vi "ReadFile.vi"(1 "Name":string="C:\\Users\\Abhi\\Documents\\test.txt") -> (0 "Array - Numeric":dbl[][](array[numeric]))   [LabVIEW 2016]
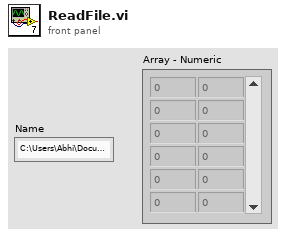
[diagram p1: front panel]
types:
  T1 = enum16{"open", "replace", "create", "open or create", "replace or create", "replace or create with confirmation"}
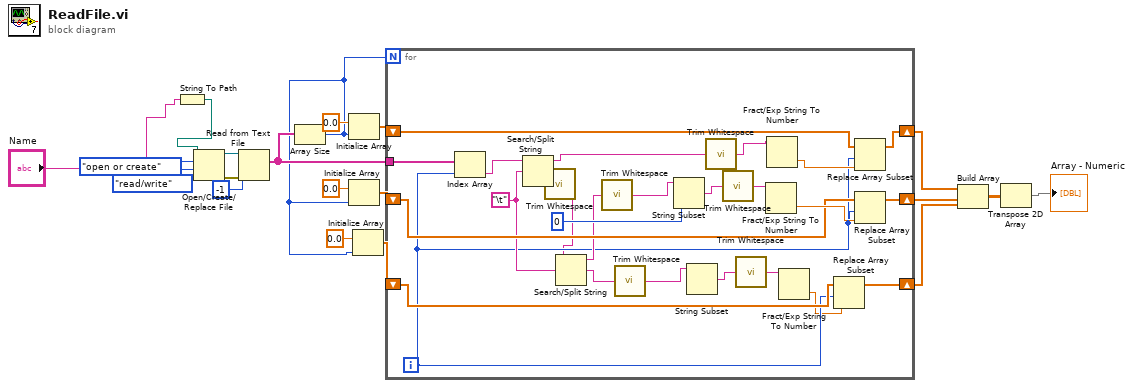
[diagram p0: block diagram]
diagram:
  n1 = String To Path(string="Name") -> (path=w6:path)
  n2 = Open/Create/Replace File(file path (use dialog)=w6, operation (0:open)=T1."open or create", access (0:read/write)=enum16{"read/write", "read-only", "write-only"}."read/write") -> (refnum out=w18:refnum<file>, error out=w17:errorcluster)  [unwired: 3 in, 1 out]
  n3 = Read from Text File(file (use dialog)=w18, count=-1, error in=w17) -> (text=w15:string[])  [unwired: 1 in, 3 out]
  n4 = Array Size(array=w15) -> (size(s)=w3:i32)
  n5 = Initialize Array(0.0 ("element"), w3) -> (w13:dbl[])
  n6 = Initialize Array(0.0 ("element"), w3) -> (w11:dbl[])
  n7 = Initialize Array(0.0 ("element"), w3) -> (w2:dbl[])
  n8 = for {
    N: w3 -> [_]
    tunnel: w15 -> [w40]
    shift-right: [w35] -> w10
    shift-left: w13 -> [w39]
    shift-right: [w34] -> w9
    shift-left: w11 -> [w36]
    shift-right: [w22] -> w1
    shift-left: w2 -> [w25]
    i -> [w24]
    w32 = "\t"
    n9 = Index Array(array=w40, index=w24) -> (element=w46:string)
    n10 = Search/Split String(string=w46, search string/char (-)=w32) -> (substring before match=w45:string, match + rest of string=w31:string)  [unwired: 1 in, 1 out]
    n11 = call <vilib>:"Trim Whitespace.vi"("string"=w31) -> ("trimmed string"=w21:string)  [unwired: 1 in]
    n12 = Search/Split String(string=w21, search string/char (-)=w32) -> (substring before match=w30:string, match + rest of string=w26:string)  [unwired: 1 in, 1 out]
    n13 = call <vilib>:"Trim Whitespace.vi"("string"=w30) -> ("trimmed string"=w33:string)  [unwired: 1 in]
    n14 = call <vilib>:"Trim Whitespace.vi"("string"=w26) -> ("trimmed string"=w27:string)  [unwired: 1 in]
    n15 = String Subset(string=w33, offset (0)=0) -> (substring=w44:string)  [unwired: 1 in]
    n16 = String Subset(string=w27) -> (substring=w29:string)  [unwired: 2 in]
    n17 = call <vilib>:"Trim Whitespace.vi"("string"=w45) -> ("trimmed string"=w42:string)  [unwired: 1 in]
    n18 = call <vilib>:"Trim Whitespace.vi"("string"=w44) -> ("trimmed string"=w41:string)  [unwired: 1 in]
    n19 = call <vilib>:"Trim Whitespace.vi"("string"=w29) -> ("trimmed string"=w28:string)  [unwired: 1 in]
    n20 = Fract/Exp String To Number(string=w41) -> (number=w37:dbl)  [unwired: 3 in, 1 out]
    n21 = Fract/Exp String To Number(string=w42) -> (number=w38:dbl)  [unwired: 3 in, 1 out]
    n22 = Fract/Exp String To Number(string=w28) -> (number=w23:dbl)  [unwired: 3 in, 1 out]
    n23 = Replace Array Subset(array=w25, new element=w23, index=w24) -> (w22:dbl[])
    n24 = Replace Array Subset(array=w39, new element=w38, index=w24) -> (w35:dbl[])
    n25 = Replace Array Subset(array=w36, new element=w37, index=w24) -> (w34:dbl[])
  }
  n26 = Build Array(w10, w9, w1) -> (w8:dbl[][])
  n27 = Transpose 2D Array(2D array=w8) -> (transposed array=→"Array - Numeric":dbl[][])
